vi "TDMSAdv getListContents.vi"(8 "error in (no error)":errorcluster, 10 "group name":string, 11 "TDMSAdv in":refnum<class "TDMSAdv.lvclass">) -> (0 "error out":errorcluster, 2 "channels":string[](array[string]), 3 "TDMSAdv out":refnum<class "TDMSAdv.lvclass">)   [LabVIEW 2018, in "TDMSAdv.lvclass"]
uses:
  TDMSAdv.lvclass
  TDMSAdv.lvclass/TDMSAdv.ctl
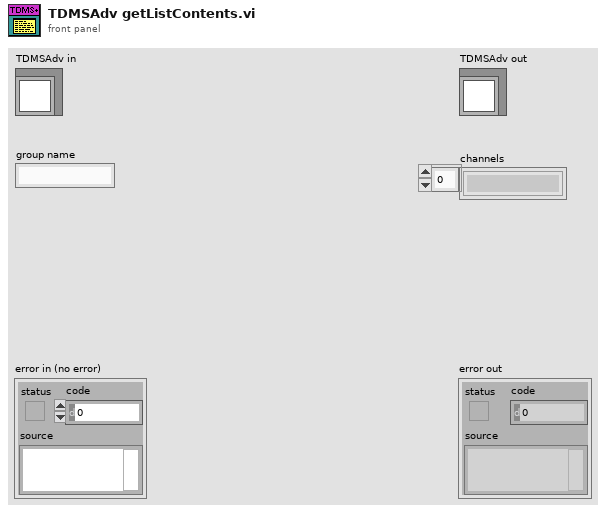
[diagram p1: front panel]
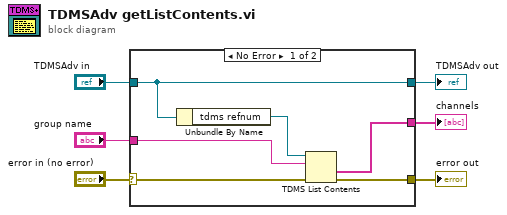
[diagram p0: block diagram]
diagram:
  n1 = case shown="No Error" "error in (no error)" {
    selector: "error in (no error)" -> [w9 w14]
    tunnel: [w8 w14] -> w5
    tunnel: [w12 w13] -> w3
    tunnel: "TDMSAdv in" -> [w12 w13]
    tunnel: "group name" -> [w10 _]
    tunnel: [w7 _] -> w1
    frame No Error {
      n2 = Unbundle By Name(w12) -> ("tdms refnum"=w11:refnum<k34>)
      n3 = TDMS List Contents(4:w9, 6:w10, 7:w11) -> (0:w8:errorcluster, 1:w7:string[])  [unwired: 2 out]
    }
    frame Error {
    }
  }
  "error out" <- w5
  "TDMSAdv out" <- w3
  "channels" <- w1
